vi "Configure Generation.vi"(8 "error in":errorcluster, 11 "DAQmx Base CFG in":refnum<class "DAQmx Base CFG.lvclass">) -> (0 "error out":errorcluster, 3 "DAQmx Base CFG out":refnum<class "DAQmx Base CFG.lvclass">)   [LabVIEW 2023, in "DAQmx Base CFG.lvclass"]
uses:
  DAQmx Base CFG.lvclass
  <vilib>/Utility/error.llb/Error Cluster From Error Code.vi
  <vilib>/ErrorRing/Error Ring.xnode
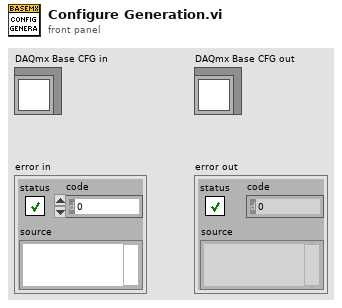
[diagram p1: front panel]
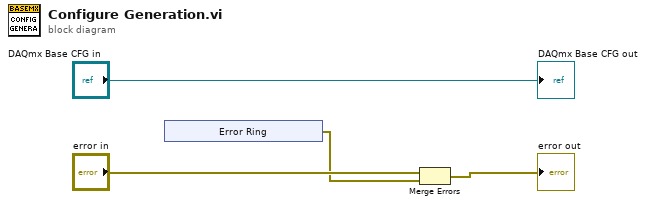
[diagram p0: block diagram]
diagram:
  n1 = xnode "Error Ring"() -> ("error out"=w1:errorcluster)
  n2 = Merge Errors("error in", w1) -> (→"error out":errorcluster)
  "DAQmx Base CFG out" <- "DAQmx Base CFG in"
